vi "Cluster Is DoubleXYData.vi"(11 "Variant":variant) -> (3 "Is DoubleXYData":bool)   [LabVIEW 2020, in "MeasurementLink Measurement Server.lvlib"]
uses:
  <vilib>/Utility/Data Type/Type Definitions/Data Type.ctl
  MeasurementLink Measurement Server.lvlib
  <vilib>/Utility/Data Type/NI_Data Type.lvlib
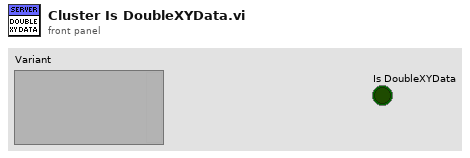
[diagram p1: front panel]
types:
  T1 = typedef "NI_Data Type.lvlib/Data Type.ctl" = enum8{"Invalid Type", "Void", "I8", "I16", "I32", "I64", "U8", "U16", "U32", "U64", "Single Float", "Double Float", "Extended Float", "Single Complex", "Double Complex", "Extended Complex", "Enum U8", "Enum U16", "Enum U32", "Enum U64", "Single Float With Unit", "Double Float With Unit", "Extended Float With Unit", "Single Complex with Unit", "Double Complex with Unit", "Extended Complex with Unit", "Boolean", "String", "Path", "Picture", "Tag", "Array", "Cluster", "Variant", "LV Variant", "Waveform", "Timestamp", "Digital Waveform", "Digital Data", "ExpressData", "Refnum", "External Data", "VI", "Poly VI", "LabVIEW Class Instance", "Fixed Point", "Set Collection", "Map Collection"}
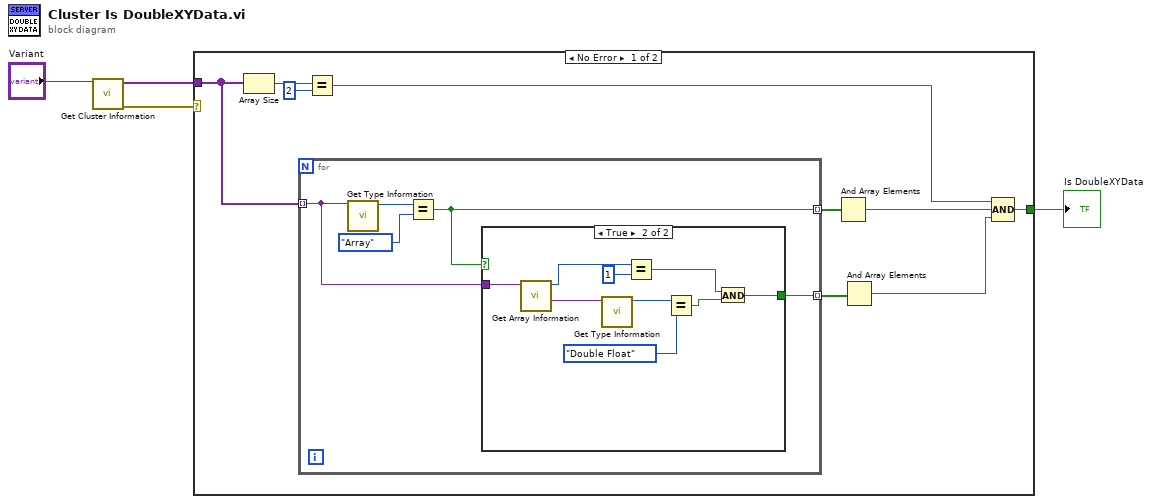
[diagram p0: block diagram]
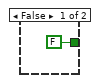
[diagram p2: hidden frame]
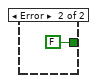
[diagram p3: hidden frame]
diagram:
  n1 = call <vilib>:"Get Cluster Information.vi"("variant"="Variant") -> ("error out"=w2:errorcluster, "cluster elements"=w4:variant[])  [unwired: 9 in]
  n2 = case shown="No Error" w2 {
    tunnel: w4 -> [w11 _]
    tunnel: [w5 FALSE] -> w3
    frame No Error {
      n3 = Array Size(array=w11) -> (size(s)=w13:i32)
      n4 = for {
        tunnel: w11 -> [w15] mode=indexing
        tunnel: [w16] -> w10 mode=indexing
        tunnel: [w14] -> w9 mode=indexing
        n5 = call <vilib>:"Get Type Information.vi"("variant"=w15) -> ("type"=w18:T1)  [unwired: 6 in, 4 out]
        n6 = Equal?(x=w18, y=Data_Type."Array") -> (x = y?=w16:bool)
        n7 = case shown="True" w16 {
          tunnel: w15 -> [_ w28]
          tunnel: [FALSE w21] -> w14
          frame False {
          }
          frame True {
            n8 = call <vilib>:"Get Array Information.vi"("variant"=w28) -> ("array element data type"=w27:variant, "number of dimensions"=w24:i32)  [unwired: 7 in, 2 out]
            n9 = call <vilib>:"Get Type Information.vi"("variant"=w27) -> ("type"=w26:T1)  [unwired: 6 in, 4 out]
            n10 = Equal?(x=w24, y=1) -> (x = y?=w22:bool)
            n11 = Equal?(x=w26, y=Data_Type."Double Float") -> (x = y?=w25:bool)
            n12 = And(x=w22, y=w25) -> (x .and. y?=w21:bool)
          }
        }
      }
      n13 = Equal?(x=w13, y=2) -> (x = y?=w8:bool)
      n14 = And Array Elements(Boolean array=w10) -> (logical AND=w7:bool)
      n15 = And Array Elements(Boolean array=w9) -> (logical AND=w6:bool)
      n16 = Compound Arithmetic op=AND(w8, w7, w6) -> (w5:bool)
    }
    frame Error {
    }
  }
  "Is DoubleXYData" <- w3
